vi "Start (Module).vi"(8 "error in (no error)":errorcluster, 9 "Module Config Element":refnum<class "VolatusConfigElement.lvclass">, 10 "Module":refnum<class "Module.lvclass">) -> (0 "error out":errorcluster, 2 "MessageQ":refnum<class "MessageQ.lvclass">)   [LabVIEW 2020, in "Volatus.lvlib" / "Volatus Core.lvclass"]
uses:
  Volatus Core.lvclass
  Volatus Core.lvclass/Volatus Core.ctl
  MessageQ/MessageQ.lvclass
  Module/Module.lvclass
  VolatusConfig/VolatusConfigElement/VolatusConfigElement.lvclass
  Top Level Module.ctl
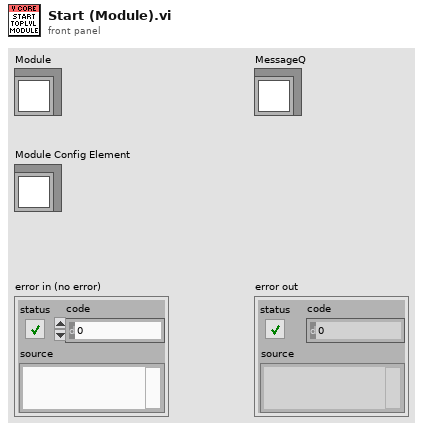
[diagram p1: front panel]
types:
  T1 = typedef "Volatus.lvlib/Volatus Core.lvclass/Top Level Module.ctl" = cluster{"Module":refnum<class "Module.lvclass">, "Config Element":refnum<class "VolatusConfigElement.lvclass">}
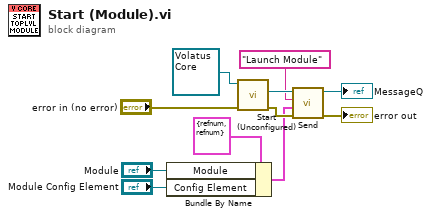
[diagram p0: block diagram]
diagram:
  n1 = Bundle By Name(cluster=T1 {"Module"=refnum, "Config Element"=refnum} ("Top Level Module"), "Module"="Module", "Config Element"="Module Config Element") -> (w1:T1)
  n2 = call "Start (Unconfigured).vi"("error in (no error)"="error in (no error)", "Volatus Core in"=refnum<class "Volatus Core.lvclass"> refnum) -> ("error out"=w6:errorcluster, "MessageQ"=w10:refnum<class "MessageQ.lvclass">)  [unwired: 8 in]
  n3 = call "Send.vi"("error in (no error)"=w6, "Data"=w1, "ID"="Launch Module", "MessageQ in"=w10) -> ("error out"=→"error out":errorcluster, "MessageQ out"=→"MessageQ":refnum<class "MessageQ.lvclass">)  [unwired: 6 in]
